vi "pressure and IK2.vi"(2 "Pressure":dbl=1.0 format="%.2f", 3 "Ft. of SS":dbl=45.0 format="%.2f", 4 "flow":dbl=10.0 format="%.2f") -> (0 "Corrected Headloss":dbl=60.584999999999994 format="%.2f", 1 "IK":dbl=0.16505735743170755 format="%.4f")   [LabVIEW 2016]
uses:
  Kpro Globals.vi
  Global_SIM_switch.vi
panel:
  out "x+y":dbl=61.8 format="%.2f"
  out "Current Depth":sgl=30.0 format="%.2f"
  out "Depth to Water Table":dbl=27.0 format="%.2f"
  out "depth out":dbl=27.0 format="%.2f"
  out "Head Loss":dbl=1.2149999999999999 format="%.2f"
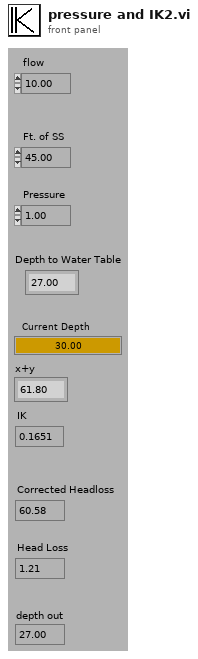
[diagram p1: front panel]
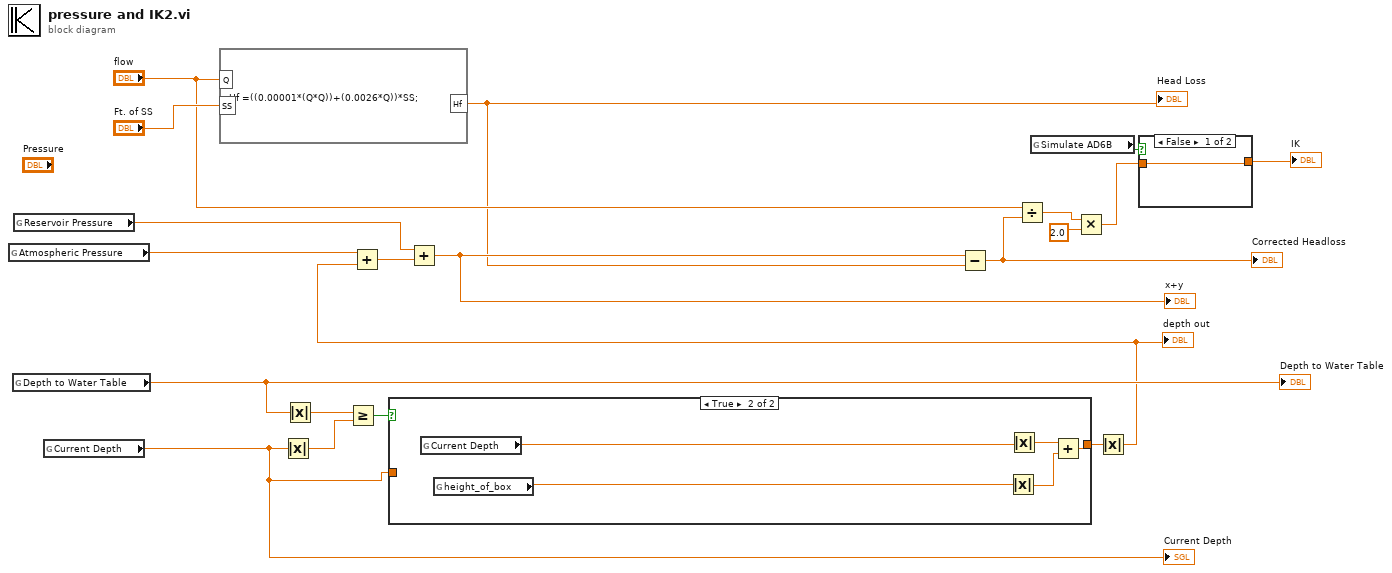
[diagram p0: block diagram]
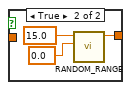
[diagram p2: hidden frame]
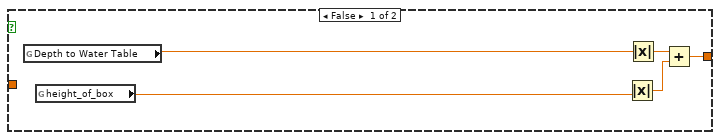
[diagram p3: hidden frame]
diagram:
  n1 = global read "Kpro Globals.vi" "Atmospheric Pressure"() -> (w15:dbl)
  n2 = global read "Kpro Globals.vi" "Depth to Water Table"() -> (w9:dbl)
  "Depth to Water Table" <- w9
  n3 = global read "Kpro Globals.vi" "Reservoir Pressure"() -> (w5:dbl)
  n4 = global read "Kpro Globals.vi" "Current Depth"() -> (w1:sgl)
  "Current Depth" <- w1
  n5 = formula code="Hf =((0.00001*(Q*Q))+(0.0026*Q))*SS;"("Q"="flow", "SS"="Ft. of SS") -> ("Hf"=w12:dbl)
  "Head Loss" <- w12
  n6 = Absolute Value(x=w1) -> (abs(x)=w8:sgl)
  n7 = Absolute Value(x=w9) -> (abs(x)=w10:dbl)
  n8 = Greater Or Equal?(x=w10, y=w8) -> (x >= y?=w16:bool)
  n9 = case shown="True" w16 {
    tunnel: [w25 w29] -> w6
    tunnel: w1 -> [_ _]
    frame False {
      n10 = global read "Kpro Globals.vi" "Depth to Water Table"() -> (w24:dbl)
      n11 = global read "Kpro Globals.vi" "height_of_box"() -> (w21:dbl)
      n12 = Absolute Value(x=w21) -> (abs(x)=w22:dbl)
      n13 = Absolute Value(x=w24) -> (abs(x)=w23:dbl)
      n14 = Add(x=w23, y=w22) -> (x+y=w25:dbl)
    }
    frame True {
      n15 = global read "Kpro Globals.vi" "Current Depth"() -> (w26:sgl)
      n16 = global read "Kpro Globals.vi" "height_of_box"() -> (w27:dbl)
      n17 = Absolute Value(x=w27) -> (abs(x)=w28:dbl)
      n18 = Absolute Value(x=w26) -> (abs(x)=w30:sgl)
      n19 = Add(x=w30, y=w28) -> (x+y=w29:dbl)
    }
  }
  n20 = global read "Global_SIM_switch.vi" "Simulate AD6B"() -> (w4:bool)
  n21 = Absolute Value(x=w6) -> (abs(x)=w7:dbl)
  "depth out" <- w7
  n22 = Add(x=w15, y=w7) -> (x+y=w14:dbl)
  n23 = Add(x=w5, y=w14) -> (x+y=w13:dbl)
  "x+y" <- w13
  n24 = Subtract(x=w13, y=w12) -> (x-y=w11:dbl)
  "Corrected Headloss" <- w11
  n25 = Divide(x="flow", y=w11) -> (x/y=w17:dbl)
  n26 = Multiply(x=w17, y=2.0) -> (x*y=w3:dbl)
  n27 = case shown="False" w4 {
    tunnel: [w31 w32] -> w2
    tunnel: w3 -> [w31 _]
    frame False {
    }
    frame True {
      n28 = call "RANDOM_RANGE.vi"("value_low"=0.0, "value_high"=15.0) -> ("Value"=w32:dbl)  [unwired: 9 in]
    }
  }
  "IK" <- w2
